vi "Camera Loop.vi"() -> ()   [LabVIEW 2011]
uses:
  <vilib>/Utility/sysdir.llb/System Directory Type.ctl
panel:
  in  "error in":errorcluster
  out "error out":errorcluster
  out "Lines":T1(array[cluster]) {"End Point"."Y" format="%.2f"; "End Point"."X" format="%.2f"; "Start Point"."Y" format="%.2f"; "Start Point"."X" format="%.2f"}
  in  "stop?":bool caption="Stop (F)"
  out "Image Out":T2(plugin-control)
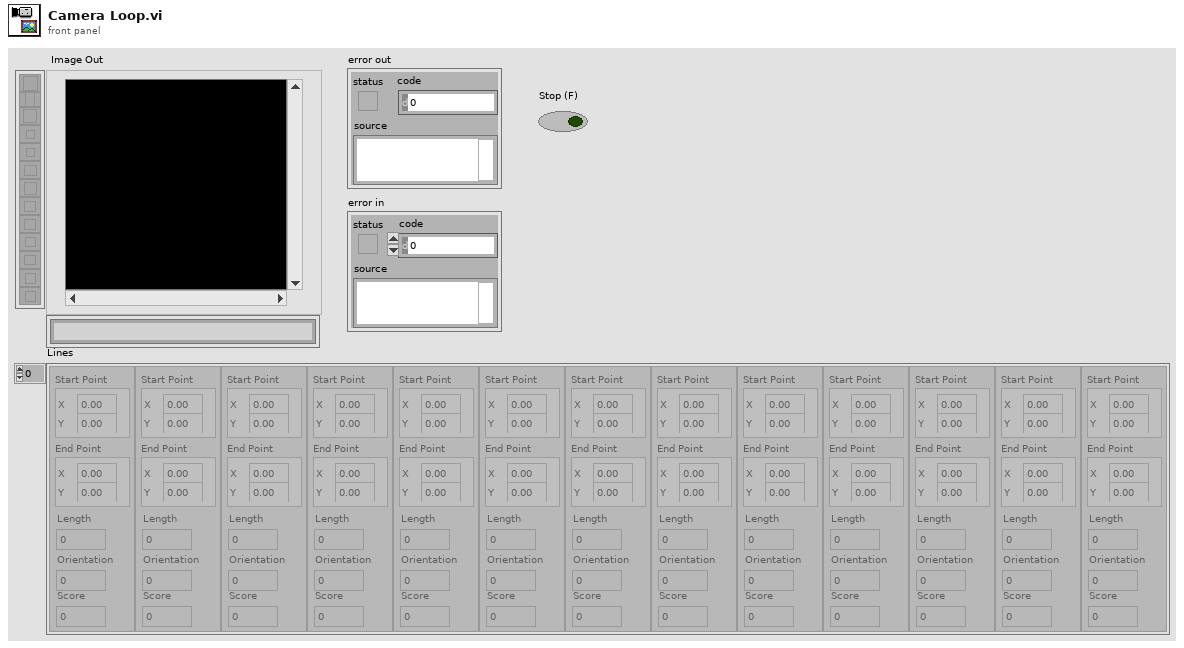
[diagram p1: front panel]
types:
  T1 = cluster{"Start Point":cluster{"X":sgl, "Y":sgl}, "End Point":cluster{"X":sgl, "Y":sgl}, "Length":dbl, "Orientation":dbl, "Score":dbl}[]
  T2 = typedef "IMAQ Image.ctl" = refnum<image>
  T3 = typedef "System Directory Type.ctl" = i32
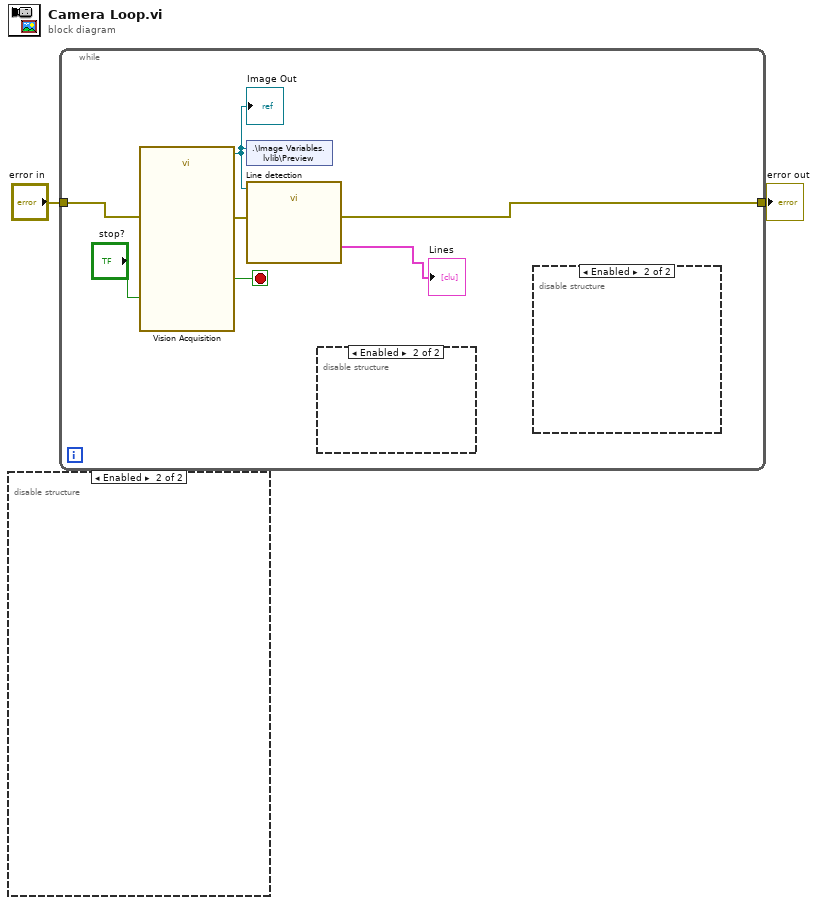
[diagram p0: block diagram]
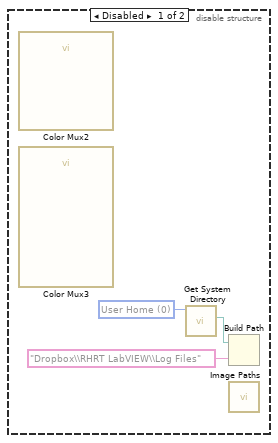
[diagram p2: hidden frame]
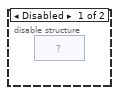
[diagram p3: hidden frame]
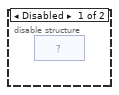
[diagram p4: hidden frame]
diagram:
  n1 = disable-structure shown="Enabled" {
    frame Disabled {
      w3 = T3 0 items=["User Home"=0, "User Desktop"=1, "User Documents"=2, "User Application Data"=3, "User Preferences"=4, "User Temporary"=5, "Public Documents"=6, "Public Application Data"=7, "Public Preferences"=8, "Public Cache"=13, "System Core Libraries"=9, "System Installed Libraries"=10, "Application Files"=11, "Boot Volume Root"=12] ("system directory type")
      n2 = call "Color Mux2"() -> ()  [unwired: 26 in, 2 out]
      n3 = call "Color Mux3"() -> ()  [unwired: 23 in, 5 out]
      n4 = call <vilib>:"Get System Directory.vi"("system directory type"=w3) -> ("system directory"=w4:path)  [unwired: 10 in]
      n5 = Build Path(base path=w4, name or relative path="Dropbox\\RHRT LabVIEW\\Log Files") -> ()  [unwired: 1 out]
      n6 = call "Image Paths.vi"() -> ()  [unwired: 10 in, 2 out]
    }
    frame Enabled {
    }
  }
  n7 = while {
    tunnel: [w7] -> w2
    tunnel: "error in" -> [w10]
    stop <- w11 stop-if-true
    n8 = call "Vision Acquisition"("Stop (F)"="stop?", "error in"=w10) -> ("Image Out"=w9:T2, "Stopped"=w11:bool, "error out"=w8:errorcluster)  [unwired: 23 in]
    "Image Out" <- w9
    n9 = shared-variable ".\\Image Variables.lvlib\\Preview"(w9) -> ()  [unwired: 1 in, 1 out]
    n10 = call "Line detection"("Image In"=w9, "error in"=w8) -> ("Lines Calibrated (Shape Detection 1)"=→"Lines":T1, "error out"=w7:errorcluster)  [unwired: 23 in, 1 out]
    n11 = disable-structure shown="Enabled" {
      frame Disabled {
        n12 = shared-variable "?"() -> ()  [unwired: 2 in, 1 out]
      }
      frame Enabled {
      }
    }
    n13 = disable-structure shown="Enabled" {
      frame Disabled {
        n14 = shared-variable "?"() -> ()  [unwired: 2 in, 1 out]
      }
      frame Enabled {
      }
    }
  }
  "error out" <- w2
